vi "AI Read.vi"(7 "AI line":T1=4000 items=["ModA/AI0"=4000, "ModA/AI1"=4001, "ModA/AI2"=4002, "ModA/AI3"=4003, "ModA/AI4"=4004, "ModA/AI5"=4005, "ModA/AI6"=4006, "ModA/AI7"=4007, "ModA/AI8"=4008, "ModA/AI9"=4009], 8 "error in (no error)":errorcluster, 11 "direct IO in":refnum<class "NI_Robotics_Starter Kit Direct IO_Sim.lvclass">) -> (0 "error out":errorcluster, 2 "data":dbl, 3 "direct IO out":refnum<class "NI_Robotics_Starter Kit Direct IO_Sim.lvclass">)   [LabVIEW 2017, in "NI_Robotics_Starter Kit Direct IO_Sim.lvclass"]
uses:
  <vilib>/robotics/Starter Kit/Sim Direct IO/NI_Robotics_Starter Kit Direct IO_Sim.lvclass
  <vilib>/robotics/Starter Kit/Direct IO/AI Lines.ctl
  <vilib>/robotics/Utilities/NI_Robotics Utilities.lvlib
  <vilib>/robotics/Starter Kit/Direct IO/NI_Robotics_Starter Kit Direct IO.lvclass
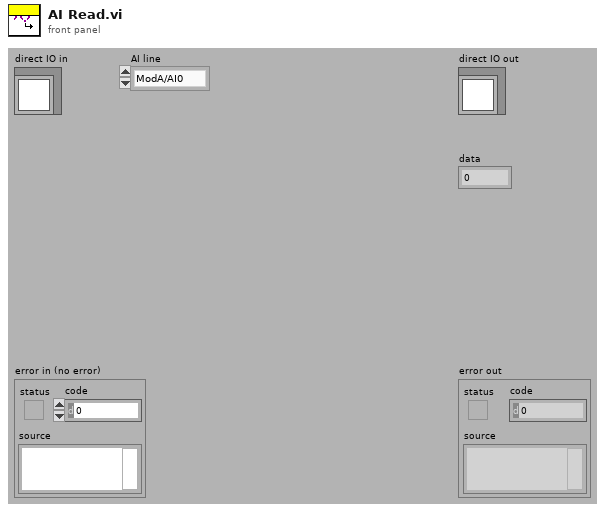
[diagram p1: front panel]
types:
  T1 = typedef "NI_Robotics_Starter Kit Direct IO.lvclass/AI Lines.ctl" = u16
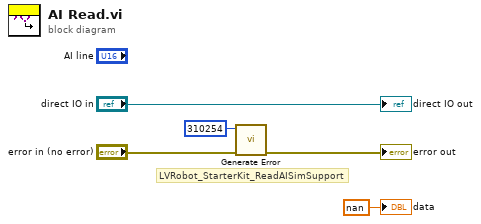
[diagram p0: block diagram]
diagram:
  # "LVRobot_StarterKit_ReadAISimSupport"
  n1 = call <vilib>:"Generate Error.vi"("error in (no error)"="error in (no error)", "code"=310254) -> ("error out"=→"error out":errorcluster)  [unwired: 9 in]
  "direct IO out" <- "direct IO in"
  "data" <- nan ("data")
